vi "Path History FG.vi"(10 "Array":i32[](array[numeric])) -> ()   [LabVIEW 2020]
panel:
  out "History":cluster{"Array":i32[]}[](array[cluster])
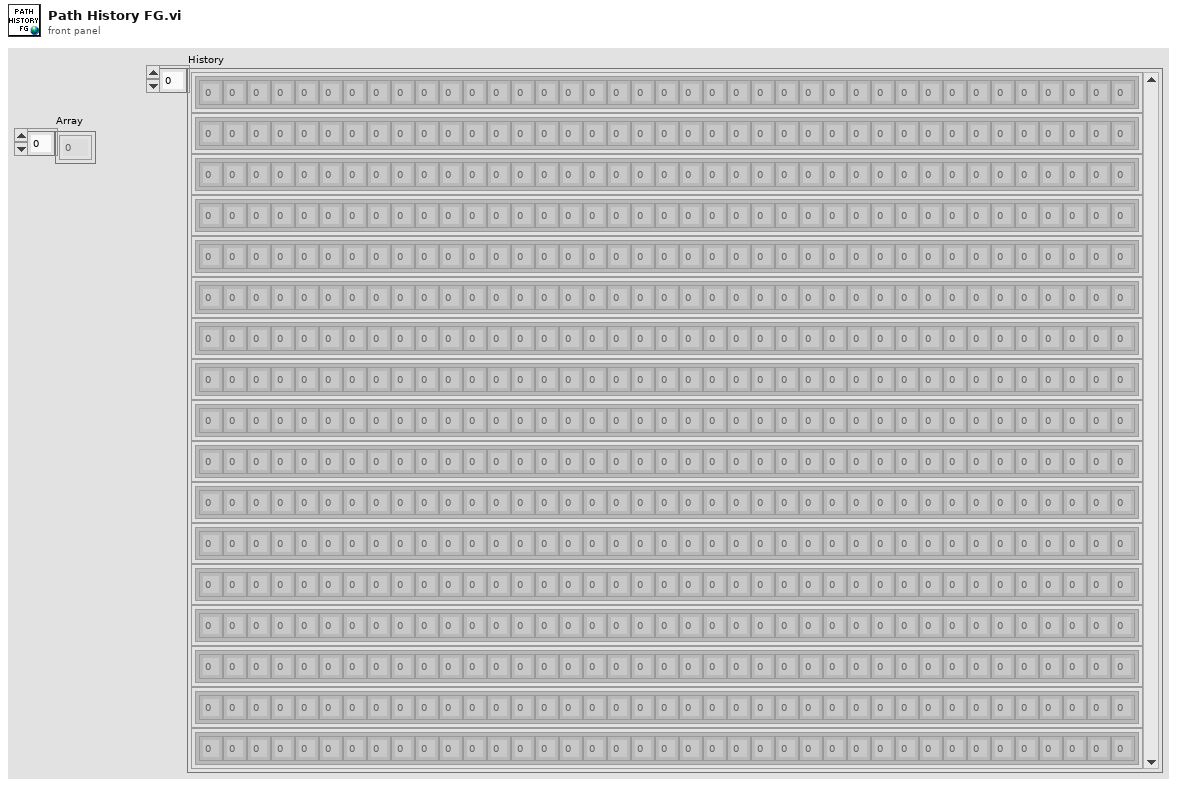
[diagram p1: front panel]
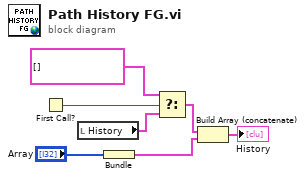
[diagram p0: block diagram]
diagram:
  n1 = First Call?() -> (First Call?: T/F=w6:bool)
  n2 = local read "History"() -> (w5:cluster{"Array":i32[]}[])
  n3 = Bundle("Array"="Array") -> (w4:cluster{"Array":i32[]})  [unwired: 1 in]
  n4 = Select(t=cluster{"Array":i32[]}[] [] ("appended array"), s=w6, f=w5) -> (s? t:f=w1:cluster{"Array":i32[]}[])
  n5 = Build Array (concatenate)(w1, w4) -> (→"History":cluster{"Array":i32[]}[])
